vi "RC_STM_Client 3.vi"() -> ()   [LabVIEW 2016, in "RemoteControl.STM.lvclass"]
uses:
  RemoteControl.STM.lvclass
  RemoteControl/RemoteControl.lvclass
  Program Files (x86)/National Instruments/LabVIEW 2019/user.lib/_OpenG.lib/numeric/numeric.llb/Random Number Within Range - I32__ogtk.vi
  Program Files (x86)/National Instruments/LabVIEW 2019/user.lib/_OpenG.lib/error/error.llb/Filter Error Codes (Array)__ogtk.vi
panel:
  in  "milliseconds to wait":u32
  out "time (1 message) (ms)":u32
  out "startup time (ms)":u32
  out "messsages/s":dbl
  in  "remote port":u16=6341
  in  "address":string
  out "Data reponse":string
  out "Messages":i32
  in  "Stop":bool
  out "Command reponse":string
  out "Command":string
  out "meta data\n(available commands)":string
  out "error out":errorcluster
  # "CLIENT (API)"
  # "Connection info"
  # "Message Sent"
  # "Message Received"
  # "Metrics"
  # "3"
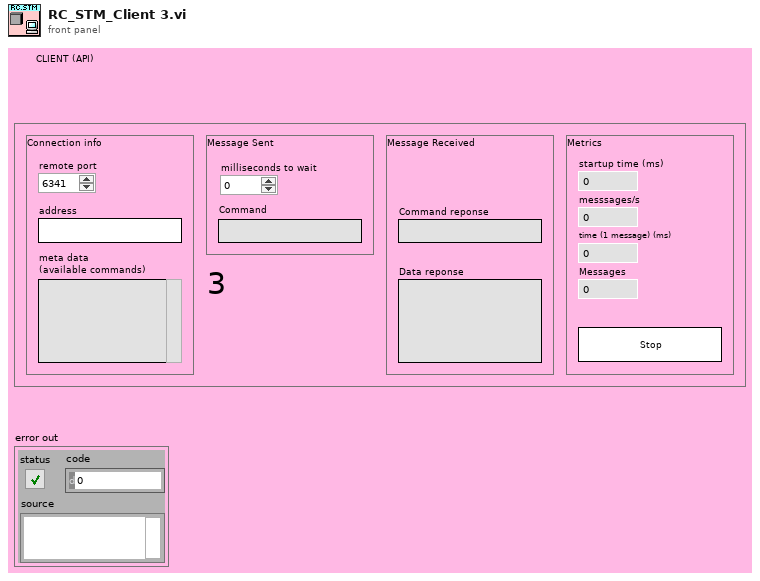
[diagram p1: front panel]
types:
  T1 = typedef "NI STM.lvlib/MetaDataElement.ctl" = string
  T2 = cluster{"Command out":string, "Data out":variant, i32}
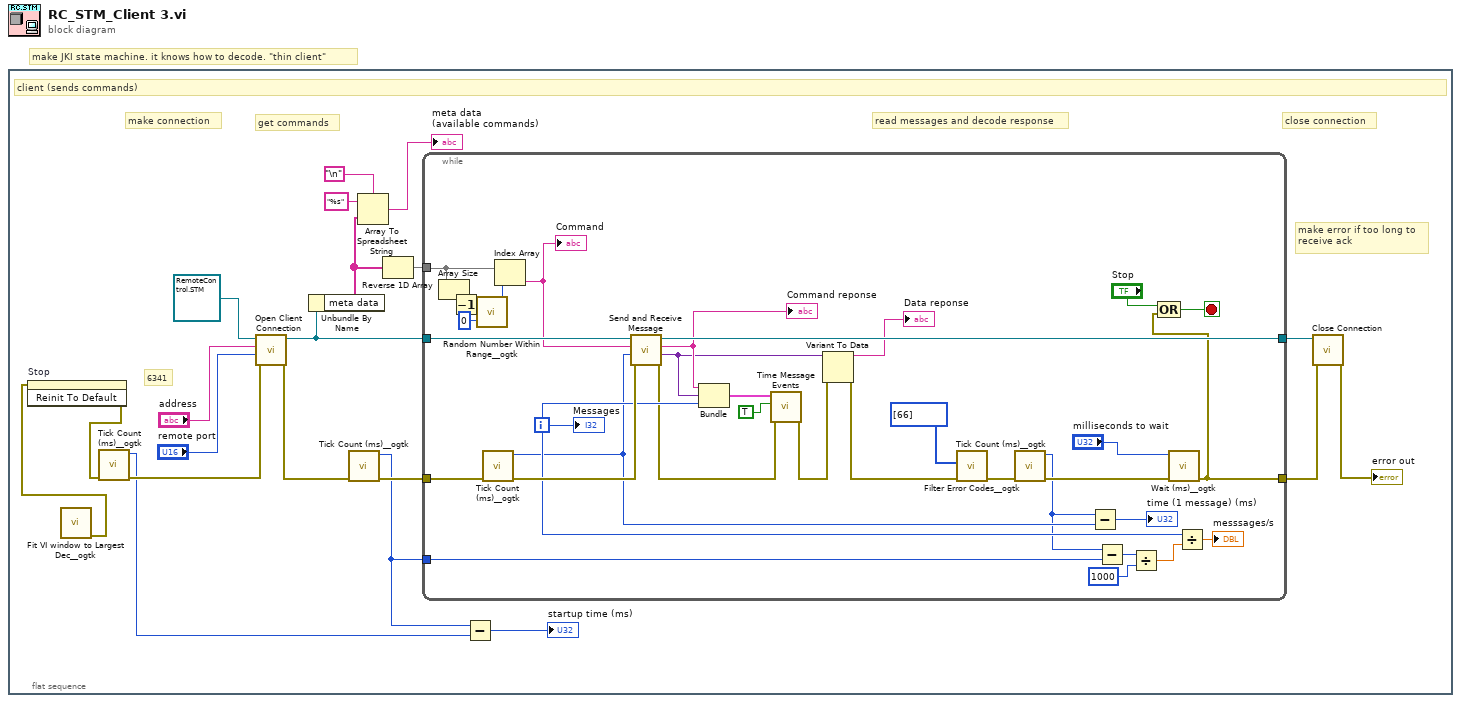
[diagram p0: block diagram]
diagram:
  # "make JKI state machine. it knows how to decode. \"thin client\""
  n1 = flat-sequence {
    frame #0 {
      # "close connection"
      # "read messages and decode response"
      # "get commands"
      # "make connection"
      # "6341"
      # "make error if too long to\nreceive ack"
      # "client (sends commands)"
      n2 = call "Fit VI window to Largest Dec__ogtk.vi"() -> ("error out"=w2:errorcluster)  [unwired: 6 in, 1 out]
      n3 = invoke on="Stop" class="Bool" method="Reinit To Default"(error in=w2) -> (error out=w18:errorcluster)  [unwired: 2 in, 2 out]
      n4 = call "Tick Count (ms)__ogtk.vi"("error in (no error)"=w18) -> ("error out"=w12:errorcluster, "millisecond timer value"=w8:u32)  [unwired: 9 in]
      n5 = call-dynamic "Open Client Connection.vi"("error in (no error)"=w12, "Port"="remote port", "address"="address", "RemoteControl.STM in"=refnum<class "RemoteControl.STM.lvclass"> refnum) -> ("error out"=w11:errorcluster, "RemoteControl.STM out"=w17:refnum<class "RemoteControl.STM.lvclass">)  [unwired: 6 in]
      n6 = Unbundle By Name(w17) -> ("meta data"=w6:T1[])
      n7 = call "Tick Count (ms)__ogtk.vi"("error in (no error)"=w11) -> ("error out"=w10:errorcluster, "millisecond timer value"=w1:u32)  [unwired: 9 in]
      n8 = Array To Spreadsheet String(delimiter (Tab)="\n", array=w6, 3:"%s" ("format string")) -> (spreadsheet string=→"meta data\n(available commands)":string)
      n9 = Reverse 1D Array(array=w6) -> (reversed array=w14:T1[])
      n10 = while {
        tunnel: [w30] -> w20
        tunnel: [w51] -> w19
        tunnel: w10 -> [w46]
        tunnel: w17 -> [w52]
        tunnel: w14 -> [w34]
        tunnel: w1 -> [w21]
        i -> [w43]
        stop <- w54 stop-if-true
        n11 = Array Size(array=w34) -> (size(s)=w35:i32)
        n12 = Decrement(x=w35) -> (x-1=w33:i32)
        n13 = call-poly "Random Number Within Range__ogtk.vi"("High"=w33, "Low"=0) -> ("Random Number"=w37:i32)  [unwired: 3 in]
        n14 = call "Tick Count (ms)__ogtk.vi"("error in (no error)"=w46) -> ("error out"=w45:errorcluster, "millisecond timer value"=w31:u32)  [unwired: 9 in]
        n15 = Index Array(array=w34, index=w37) -> (element=w47:T1)
        "Command" <- w47
        n16 = call-dynamic "Send and Receive Message.vi"("error in (no error)"=w45, "Data"=w31, "Command"=w47, "RemoteControl in"=w52) -> ("error out"=w32:errorcluster, "Data out"=w29:variant, "Command out"=w44:string, "RemoteControl out"=w51:refnum<class "RemoteControl.STM.lvclass">)  [unwired: 4 in]
        "Command reponse" <- w44
        n17 = Bundle("Command out"=w44, "Data out"=w29, w43) -> (w42:T2)  [unwired: 1 in]
        n18 = call "Time Message Events.vi"("error in (no error)"=w32, "Debug Mode"=TRUE, "Message in"=w42) -> ("error out"=w28:errorcluster)  [unwired: 6 in, 2 out]
        n19 = Variant To Data(error in=w28, Variant=w29) -> (data=→"Data reponse":string, error out=w27:errorcluster)  [unwired: 1 in]
        n20 = call-poly "Filter Error Codes__ogtk.vi"("Error In"=w27, "Error Codes to Filter"=i32[] [66]) -> ("Error Out"=w50:errorcluster)  [unwired: 7 in, 2 out]
        n21 = call "Tick Count (ms)__ogtk.vi"("error in (no error)"=w50) -> ("error out"=w40:errorcluster, "millisecond timer value"=w23:u32)  [unwired: 9 in]
        n22 = Subtract(x=w23, y=w31) -> (x-y=→"time (1 message) (ms)":u32)
        n23 = Subtract(x=w23, y=w21) -> (x-y=w22:u32)
        n24 = Divide(x=w22, y=u32 1000) -> (x/y=w49:dbl)
        n25 = call "Wait (ms)__ogtk.vi"("error in (no error)"=w40, "milliseconds to wait"="milliseconds to wait") -> ("error out"=w30:errorcluster)  [unwired: 8 in, 1 out]
        n26 = Compound Arithmetic op=OR("Stop", w30) -> (w54:bool)
        n27 = Divide(x=w43, y=w49) -> (x/y=→"messsages/s":dbl)
        "Messages" <- w43
      }
      n28 = Subtract(x=w1, y=w8) -> (x-y=→"startup time (ms)":u32)
      n29 = call-dynamic "Close Connection.vi"("error in (no error)"=w20, "RemoteControl.STM in"=w19) -> ("error out"=→"error out":errorcluster)  [unwired: 8 in, 1 out]
    }
  }
